vi "Engage_Switch.vi"(8 "error in (no error)":errorcluster, 10 "Parameters":string, 11 "reference in":refnum<class "Test_NanoP5.lvclass">) -> (0 "error out":errorcluster, 2 "Result":bool, 3 "reference out":refnum<class "Test_NanoP5.lvclass">)   [LabVIEW 2019]
uses:
  Test_NanoP5.lvclass
  Components/SwitchBase.lvlibp/SwitchBase.lvclass
  <vilib>/addons/_JKI.lib/Serialization/JSON/JKI JSON Serialization.lvlib
  ParameterTypes/PowerDUT.ctl
panel:
  in  "Parameter_Type":T1
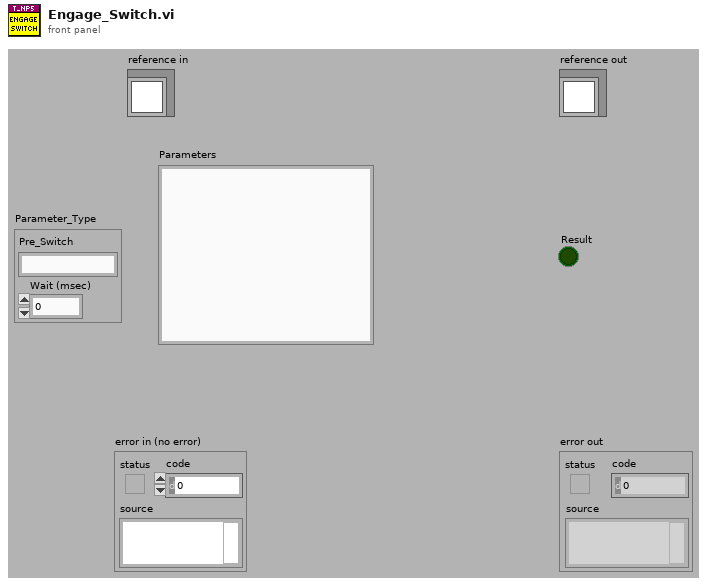
[diagram p1: front panel]
types:
  T1 = typedef "Test_NanoP5.lvlib/Test_NanoP5.lvclass/PowerDUT.ctl" = cluster{"Pre_Switch":string, "Wait (msec)":i32}
  T2 = typedef "Test_NanoP5.lvlib/Test_NanoP5.lvclass/ObjectAttributes.ctl" = cluster{"Config":T3, "DMM":refnum<class "DMM_Keysight_34980A.lvclass">, "LCR":refnum<class "LCR_BK891.lvclass">, "PSU":refnum<class "PSU_Base.lvclass">, "Switch_Manager":refnum<class "SwitchBase.lvclass">, "Switch_Motor":refnum<class "SwitchBase.lvclass">, "NanoP5":refnum<class "NanoP5.lvclass">}
  T3 = typedef "Test_NanoP5.lvlib/Test_NanoP5.lvclass/Config.ctl" = cluster{"default":string}
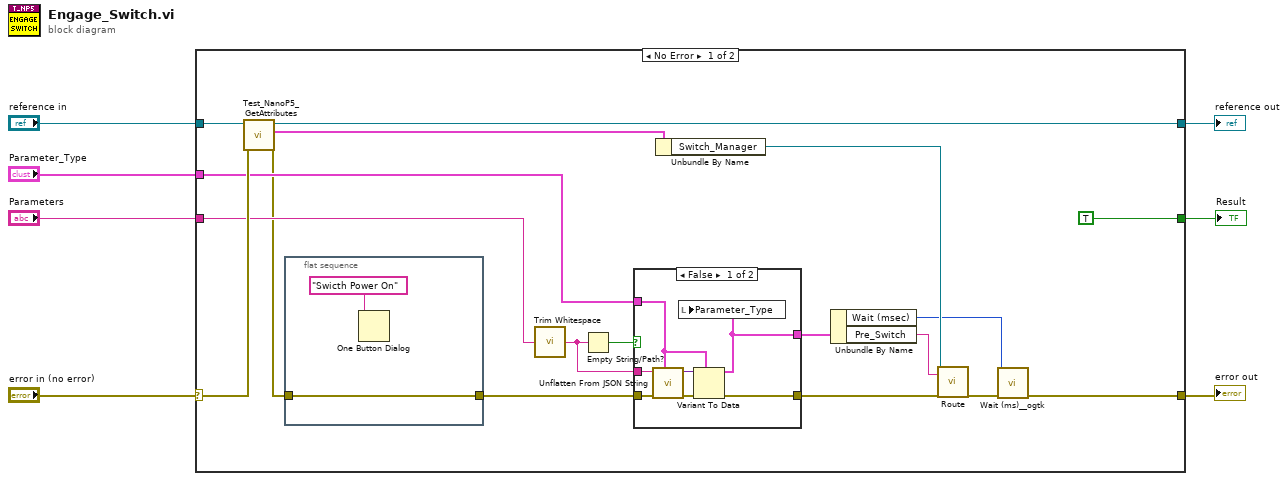
[diagram p0: block diagram]
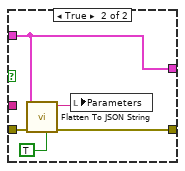
[diagram p2: hidden frame]
diagram:
  n1 = case shown="No Error" "error in (no error)" {
    selector: "error in (no error)" -> [w25 w41]
    tunnel: [w11 w41] -> w6
    tunnel: [w23 w40] -> w4
    tunnel: "reference in" -> [w24 w40]
    tunnel: "Parameters" -> [w16 _]
    tunnel: "Parameter_Type" -> [w17 _]
    tunnel: [TRUE _] -> w1
    frame No Error {
      n2 = call "Test_NanoP5_GetAttributes.vi"("error in (no error)"=w25, "reference in"=w24) -> ("error out"=w9:errorcluster, "Data"=w22:T2, "reference out"=w23:refnum<class "Test_NanoP5.lvclass">)  [unwired: 6 in, 1 out]
      n3 = flat-sequence {
        tunnel: w9 -> [w27]
        tunnel: [w27] -> w8
        frame #0 {
          n4 = One Button Dialog(message="Swicth Power On") -> ()  [unwired: 1 in, 1 out]
        }
      }
      n5 = call <vilib>:"Trim Whitespace.vi"("string"=w16) -> ("trimmed string"=w19:string)  [unwired: 1 in]
      n6 = Empty String/Path?(string/path=w19) -> (empty?=w18:bool)
      n7 = case shown="False" w18 {
        tunnel: w8 -> [w32 w38]
        tunnel: w17 -> [w31 w37]
        tunnel: [w30 w39] -> w12
        tunnel: [w28 w37] -> w15
        tunnel: w19 -> [w29 _]
        frame False {
          n8 = call <vilib>:"Unflatten From JSON String.vi"("Type and Defaults"=w31, "error in (no error)"=w32, "JSON String"=w29) -> ("error out"=w34:errorcluster, "Variant"=w33:variant)  [unwired: 7 in]
          n9 = Variant To Data(error in=w34, type=w31, Variant=w33) -> (data=w28:T1, error out=w30:errorcluster)
          n10 = local write "Parameter_Type"(w28) -> ()
        }
        frame True {
          n11 = call <vilib>:"Flatten To JSON String.vi"("Enums As String (F)"=TRUE, "error in (no error)"=w38, "Variant"=w37) -> ("error out"=w39:errorcluster, "JSON String"=w36:string)  [unwired: 7 in]
          n12 = local write "Parameters"(w36) -> ()
        }
      }
      n13 = Unbundle By Name(w22) -> ("Switch_Manager"=w21:refnum<class "SwitchBase.lvclass">)
      n14 = Unbundle By Name(w15) -> ("Wait (msec)"=w13:i32, "Pre_Switch"=w14:string)
      n15 = call-dynamic "Route.vi"("reference in"=w21, "channel 1"=w14, "error in (no error)"=w12) -> ("error out"=w20:errorcluster)  [unwired: 15 in, 1 out]
      n16 = call <userlib>:"Wait (ms)__ogtk.vi"("error in (no error)"=w20, "milliseconds to wait"=w13) -> ("error out"=w11:errorcluster)  [unwired: 8 in, 1 out]
    }
    frame Error {
    }
  }
  "Result" <- w1
  "error out" <- w6
  "reference out" <- w4
